vi "getImgAttributesFromTree.vi"(8 "error in (no error)":errorcluster, 9 "Cluster in":T1, 10 "Tree pics & devs in":string, 11 "TreeControl in":refnum<vi>) -> (0 "error out":errorcluster, 3 "Cluster out":T1)   [LabVIEW 2013, in "TreeRepresentation.lvlib"]
uses:
  TreeRepresentation.lvlib
  vis/SetupData2.ctl
  classes/Datastructure/Device/Device.lvclass
  classes/Datastructure/Image/img.lvclass
  DataCreation.lvlib
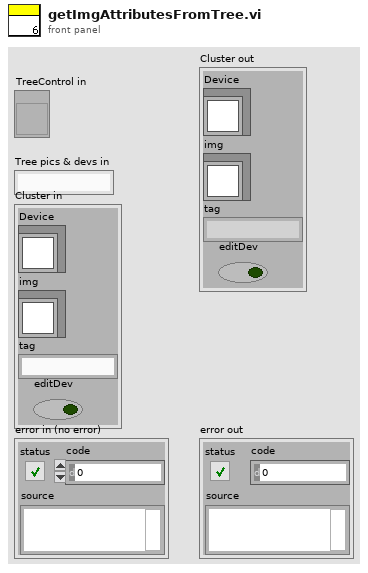
[diagram p1: front panel]
types:
  T1 = typedef "DataCreation.lvlib/SetupData2.ctl" = cluster{"Device":refnum<class "Device.lvclass">, "img":refnum<class "img.lvclass">, "tag":string, "editDev":bool}
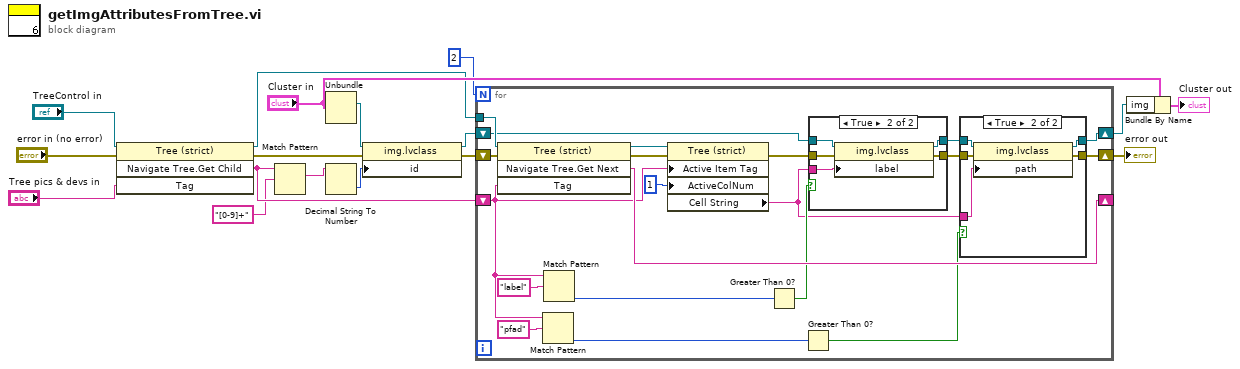
[diagram p0: block diagram]
diagram:
  n1 = invoke class="Tree (strict)" method="Navigate Tree.Get Child"(reference="TreeControl in", error in="error in (no error)", "Tag"="Tree pics & devs in") -> (reference out=w11:refnum<vi>, error out=w6:errorcluster, "Navigate Tree:Get Child"=w4:string)  [unwired: 1 in, 1 out]
  n2 = Match Pattern(string=w4, regular expression="[0-9]+") -> (match substring=w2:string)  [unwired: 1 in, 3 out]
  n3 = Unbundle("Cluster in") -> ("img"=w8:refnum<class "img.lvclass">)  [unwired: 3 out]
  n4 = Decimal String To Number(string=w2) -> (number=w1:i32)  [unwired: 2 in, 1 out]
  n5 = property class="img.lvclass"(reference=w8, error in=w6, "id"=w1) -> (reference out=w7:refnum<class "img.lvclass">, error out=w5:errorcluster)
  n6 = for {
    N: 2 -> [_]
    tunnel: w11 -> [w28]
    shift-right: [w37] -> _
    shift-left: w4 -> [w33]
    shift-right: [w23] -> w16
    shift-left: w5 -> [w29]
    shift-right: [w22] -> w15
    shift-left: w7 -> [w19]
    n7 = invoke class="Tree (strict)" method="Navigate Tree.Get Next"(reference=w28, error in=w29, "Tag"=w33) -> (reference out=w24:refnum<vi>, error out=w26:errorcluster, "Navigate Tree:Get Next Item"=w37:string)  [unwired: 1 in, 1 out]
    n8 = Match Pattern(string=w33, regular expression="pfad") -> (offset past match=w34:i32)  [unwired: 1 in, 3 out]
    n9 = Match Pattern(string=w33, regular expression="label" ("Left Cell String")) -> (offset past match=w35:i32)  [unwired: 1 in, 3 out]
    n10 = property class="Tree (strict)"(reference=w24, error in=w26, "Active Item Tag"=w33, "ActiveColNum"=1 ("Active Cell:Active Column Number")) -> (error out=w18:errorcluster, "Cell String"=w25:string)  [unwired: 1 out]
    n11 = Greater Than 0?(x=w35) -> (x > 0?=w32:bool)
    n12 = Greater Than 0?(x=w34) -> (x > 0?=w31:bool)
    n13 = case shown="True" w32 {
      tunnel: w18 -> [w45 w51]
      tunnel: [w45 w50] -> w27
      tunnel: w19 -> [w46 w49]
      tunnel: [w46 w48] -> w30
      tunnel: w25 -> [_ w47]
      frame False {
      }
      frame True {
        n14 = property class="img.lvclass"(reference=w49, error in=w51, "label"=w47) -> (reference out=w48:refnum<class "img.lvclass">, error out=w50:errorcluster)
      }
    }
    n15 = case shown="True" w31 {
      tunnel: w27 -> [w38 w44]
      tunnel: [w38 w43] -> w23
      tunnel: w30 -> [w39 w42]
      tunnel: [w39 w41] -> w22
      tunnel: w25 -> [_ w40]
      frame False {
      }
      frame True {
        n16 = property class="img.lvclass"(reference=w42, error in=w44, "path"=w40) -> (reference out=w41:refnum<class "img.lvclass">, error out=w43:errorcluster)
      }
    }
  }
  "error out" <- w16
  n17 = Bundle By Name(cluster="Cluster in", "img"=w15) -> (→"Cluster out":T1)
